vi "SV Convert Spectra to Data Object.vi"(0 "spectra":cluster{"f0":dbl, "df":dbl, "magnitude":dbl[]}[](array[cluster]) {"magnitude" format="%.2p"; "df" format="%.2p"; "f0" format="%.2p"}, 4 "spectra info":T1[](array[typedef]) {"x-axis units" items=["Time (s)"=0, "Frequency-CB (Hz)"=1, "Frequency-CPB (Hz)"=1248, "Frequency-Arbitrary (Hz)"=2357, "Quefrency (s)"=2, "Revolutions (rev)"=3, "Order"=4, "Speed (RPM)"=11, "Speed (rad/s)"=21, "Index"=65535]; "weighting filter" items=["Linear", "A-weighting", "B-weighting", "C-weighting", "ITU-R 468-4", "Dolby", "CCITT", "C-message", "Wb", "Wc", "Wd", "We", "Wf", "Wh", "Wj", "Wk", "Wm", "AES17 20 kHz lowpass", "AES17 40 kHz lowpass", "AES17 20 kHz highpass", "AES17 40 kHz highpass"]; "dB reference [EU]" format="%.2f"; "engineering units" items=["custom..."=0, "V"=1, "A"=21, "C"=30, "pC"=31, "s"=32, "-"=29, "Pa"=2, "N"=20, "g"=3, "m/s^2"=4, "m/s"=5, "m"=6, "mm/s"=12, "mm"=13, "micron/s"=14, "micron"=15, "in/s^2"=7, "in/s"=8, "in"=9, "mil/s"=10, "mil"=11, "rad/s^2"=16, "rad/s"=17, "rad"=18, "deg/s^2"=26, "deg/s"=27, "deg"=28, "RPM"=22, "cycle/s^2"=23, "Hz"=24, "cycle"=25, "strain"=19]; "spectral info"."window" items=["None "=0, "Hanning"=1, "Hamming"=2, "Blackman-Harris"=3, "Exact Blackman"=4, "Blackman"=5, "Flat Top"=6, "4 Term B-Harris "=7, "7 Term B-Harris"=8, "Low Sidelobe"=9, "Force - Exponential"=10, "Gaussian"=62]}, 5 "error in (no error)":errorcluster) -> (14 "Spectrum Data":refnum<class "Data.lvclass">, 19 "error out":errorcluster)   [LabVIEW 2017, in "Y (N Ch).lvclass"]
doc: "Use this polymorphic VI to convert spectra to a class data type that you can view on the Spectrum with Cursors XControl. You must manually select the polymorphic instance to use."
uses:
  <vilib>/addons/_NISVFA/_Shared subVIs/Data Objects/Y (DBL)/Y (N Ch).lvclass
  <vilib>/addons/_NISVFA/_Shared subVIs/Controls/svc_Spectrum Info.ctl
  <vilib>/addons/_NISVFA/_Shared subVIs/Controls/svc_X-Axis Units.ctl
  <vilib>/addons/_NISVFA/_Shared subVIs/Controls/svc_Spectrum Type.ctl
  <vilib>/addons/_NISVFA/_Shared subVIs/Controls/svc_Engineering Units Text Ring.ctl
  <vilib>/addons/_NISVFA/_Shared subVIs/Controls/svc_Weighting Filter Text Ring.ctl
  <vilib>/addons/_NISVFA/_Shared subVIs/Controls/svc_Complimentary Spectrum Units.ctl
  <vilib>/addons/_NISVFA/_Shared subVIs/Data Objects/Data/Data.lvclass
  C:/Program Files (x86)/National Instruments/LabVIEW 2017/vi.lib/addons/_NISVFA/_Shared subVIs/Data Objects/Data/Data.lvclass
  <vilib>/addons/_NISVFA/_Shared subVIs/Controls/NI Channel Properties.ctl
  <vilib>/addons/_NISVFA/_Shared subVIs/Data Objects/Y (DBL)/Y (N Ch).lvclass/Y (N Ch).ctl
  <vilib>/addons/_NISVFA/_Shared subVIs/Data Objects/Data/Data.lvclass/Data.ctl
  <vilib>/addons/_NISVFA/_Shared subVIs/Data Objects/Data/Read Data Attributes.vi
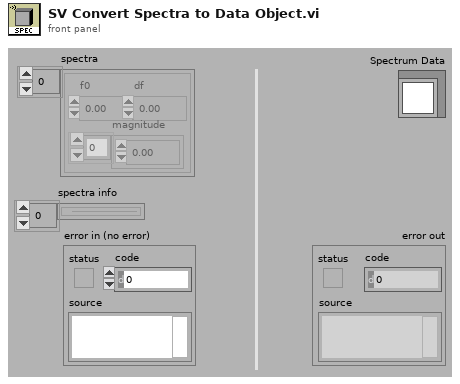
[diagram p1: front panel]
types:
  T1 = typedef "svc_Spectrum Info.ctl" = cluster{"channel name":string, "description":string, "x-axis units":T2, "spectral info":cluster{"spectrum type":T3, "linear/dB":enum16{"linear", "dB"}, "window":u16, "window size":i32, "FFT size":i32}, "engineering units":T4, "custom label":string, "dB reference [EU]":dbl, "peak units":enum16{"rms", "peak", "peak-peak"}, "weighting filter":T5, "spectral density?":bool, "unit label":string, "spectrum skewed?":bool, "complimentary spectrum units":T6}
  T2 = typedef "svc_X-Axis Units.ctl" = u16
  T3 = typedef "svc_Spectrum Type.ctl" = enum16{"FFT Spectrum [complex]", "Amplitude [Magnitude]", "Power [Magnitude^2]", "Cross Spectrum [complex]", "Frequency Response [Complex]"}
  T4 = typedef "svc_Engineering Units Text Ring.ctl" = u16
  T5 = typedef "svc_Weighting Filter Text Ring.ctl" = u16
  T6 = typedef "svc_Complimentary Spectrum Units.ctl" = enum16{"none", "radians", "degrees", "cycles", "imaginary"}
  T7 = cluster{"Y":dbl[], "channel attributes":variant}[]
  T8 = typedef "NI Channel Properties.ctl" = u16
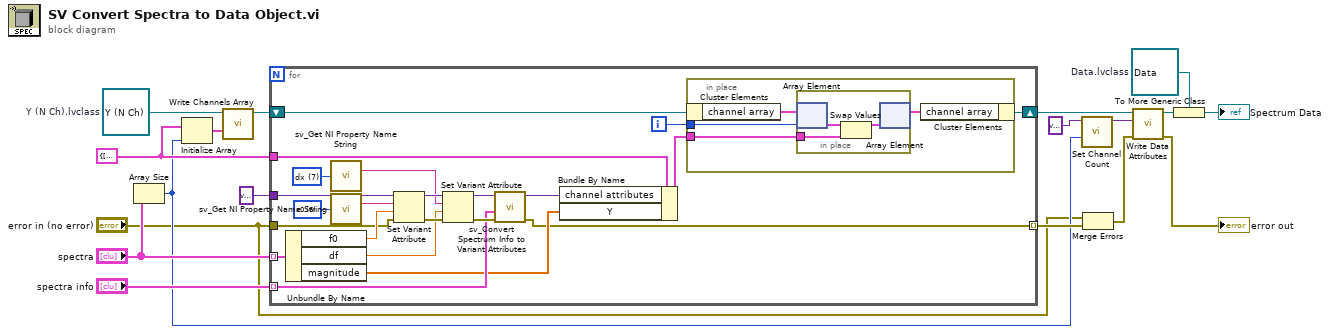
[diagram p0: block diagram]
diagram:
  w10 = cluster{"Y":dbl[], "channel attributes":variant} {"Y"=[], "channel attributes"=variant} ("channel data")
  w17 = refnum<class "Data.lvclass"> refnum  # Data.lvclass
  w7 = refnum<class "Y (N Ch).lvclass"> refnum  # Y (N Ch).lvclass
  n1 = Array Size(array="spectra") -> (size(s)=w2:i32)
  n2 = Initialize Array(w10, w2) -> (w8:T7)
  n3 = call <vilib>:"Write Channels Array.vi"("channel array"=w8, "Y (N Ch) in"=w7) -> ("Y (N Ch) out"=w6:refnum<class "Y (N Ch).lvclass">)  [unwired: 8 in, 1 out]
  n4 = for {
    tunnel: "spectra" -> [w40] mode=indexing
    tunnel: "spectra info" -> [w33] mode=indexing
    tunnel: variant ("data attributes") -> [w28]
    tunnel: w10 -> [w27]
    tunnel: "error in (no error)" -> [w24]
    tunnel: [w23] -> w12 mode=indexing
    shift-right: [w19] -> w5
    shift-left: w6 -> [w20]
    i -> [w22]
    w31 = T8 6 items=["Channel name", "Channel description", "Axis label", "Unit string", "Waveform X-axis label", "Waveform X-axis unit string", "x0", "dx", "Number of samples", "X channel", "Filter settled", "dB reference", "Window", "Window parameter", "Window size", "FFT size", "Peak units", "Spectrum type", "Magnitude scale", "Spectral density", "Sensor sensitivity (mV/EU)", "X-axis dimension", "LabVIEW datatype", "Function type", "Function subtype", "X values", "Independent channel", "Column index", "Collection name", "Collection ID", "X Columns", "Phase unwrapped"] ("property")
    w32 = T8 7 items=["Channel name", "Channel description", "Axis label", "Unit string", "Waveform X-axis label", "Waveform X-axis unit string", "x0", "dx", "Number of samples", "X channel", "Filter settled", "dB reference", "Window", "Window parameter", "Window size", "FFT size", "Peak units", "Spectrum type", "Magnitude scale", "Spectral density", "Sensor sensitivity (mV/EU)", "X-axis dimension", "LabVIEW datatype", "Function type", "Function subtype", "X values", "Independent channel", "Column index", "Collection name", "Collection ID", "X Columns", "Phase unwrapped"] ("property")
    n5 = Unbundle By Name(w40) -> ("f0"=w35:dbl, "df"=w34:dbl, "magnitude"=w25:dbl[])
    n6 = call <vilib>:"sv_Get NI Property Name String.vi"("property"=w32) -> ("TDMS property name"=w29:string)  [unwired: 13 in, 1 out]
    n7 = call <vilib>:"sv_Get NI Property Name String.vi"("property"=w31) -> ("TDMS property name"=w30:string)  [unwired: 13 in, 1 out]
    n8 = Set Variant Attribute(Variant=w28, name=w30, value=w35, error in=w24) -> (Variant out=w37:variant, error out=w38:errorcluster)  [unwired: 1 out]
    n9 = Set Variant Attribute(Variant=w37, name=w29, value=w34, error in=w38) -> (Variant out=w39:variant, error out=w36:errorcluster)  [unwired: 1 out]
    n10 = call <vilib>:"sv_Convert Spectrum Info to Variant Attributes.vi"("error in"=w36, "spectrum info"=w33, "attributes in"=w39) -> ("error out"=w23:errorcluster, "attributes out"=w26:variant)  [unwired: 5 in, 2 out]
    n11 = Bundle By Name(cluster=w27, "channel attributes"=w26, "Y"=w25) -> (w21:cluster{"Y":dbl[], "channel attributes":variant})
    n12 = in-place {
      in-place-border: w22 -> [w43]
      in-place-border: w21 -> [w41]
      n13 = in-place-cluster #1(w20) -> ("channel array"=w44:T7)
      n14 = in-place {
        in-place-border: w41 -> [w45]
        n15 = in-place-array #2(w44, w43) -> (w47:cluster{"Y":dbl[], "channel attributes":variant})
        n16 = Swap Values(12:w47, 14:w45) -> (1:w46:cluster{"Y":dbl[], "channel attributes":variant})  [unwired: 1 in, 1 out]
        n17 = in-place-array #2(w46) -> (w42:T7)  [unwired: 1 out]
      }
      n18 = in-place-cluster #1("channel array"=w42) -> (w19:refnum<class "Y (N Ch).lvclass">)
    }
  }
  n19 = call <vilib>:"Set Channel Count.vi"("number of channels"=w2, "variant in"=variant ("data attributes")) -> ("variant out"=w3:variant)  [unwired: 9 in]
  n20 = Merge Errors("error in (no error)", w12) -> (w11:errorcluster)
  n21 = call <vilib>:"Write Data Attributes.vi"("error in (no error)"=w11, "data attributes"=w3, "Data in"=w5) -> ("error out"=→"error out":errorcluster, "Data out"=w14:refnum<class "Y (N Ch).lvclass">)  [unwired: 7 in]
  n22 = To More Generic Class(target class=w17, reference=w14) -> (generic class reference=→"Spectrum Data":refnum<class "Data.lvclass">)
